vi "Alerte_Temperature (Sub) icon test.vi"() -> ()   [LabVIEW 2024]
panel:
  out "Message d'Alerte":string
  out "Avertissement?":bool
  in  "Temp Min":dbl
  in  "Temp Max":dbl
  in  "Temp":dbl
  # "TP N°2"
  # "Mekni Marwen 2ème Année Génie Electrique"
  # "Icon Test"
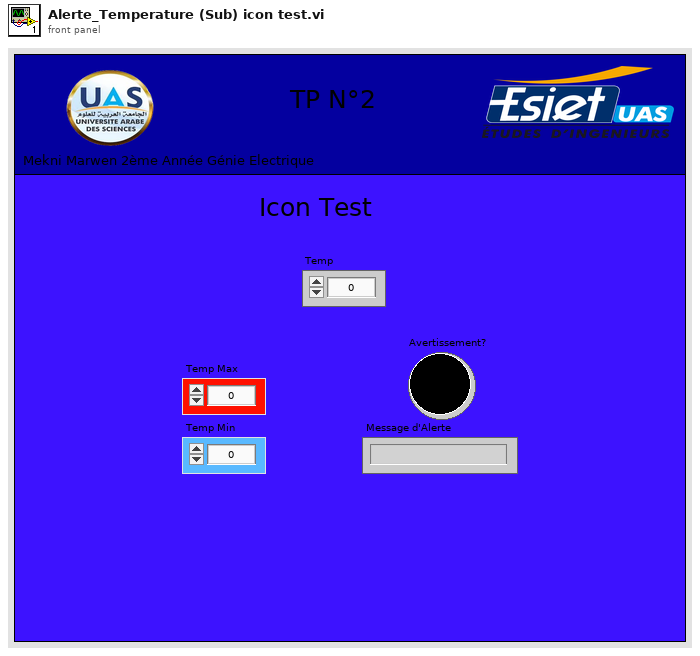
[diagram p1: front panel]
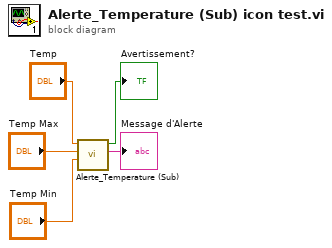
[diagram p0: block diagram]
diagram:
  n1 = call "Alerte_Temperature (Sub).vi"("Temp Min"="Temp Min", "Temp Max"="Temp Max", "Temp"="Temp") -> ("Message d'Alerte"=→"Message d'Alerte":string, "Avertissement?"=→"Avertissement?":bool)  [unwired: 6 in, 1 out]
